vi "stopReading.vi"(8 "error in (no error)":errorcluster, 10 "Electrometer in":refnum<class "Electrometer.lvclass">, 11 "State in":refnum<class "State.lvclass">) -> (0 "error out":errorcluster, 2 "Electrometer out":refnum<class "Electrometer.lvclass">, 3 "State out":refnum<class "State.lvclass">)   [LabVIEW 2016, in "State.lvclass"]
uses:
  State.lvclass
  Electrometer.lvclass
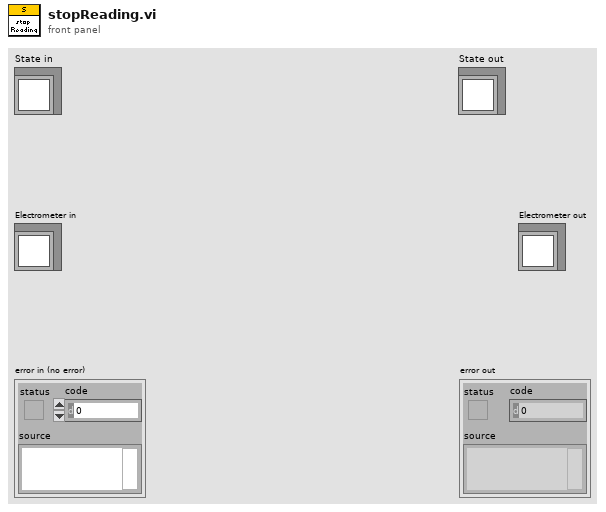
[diagram p1: front panel]
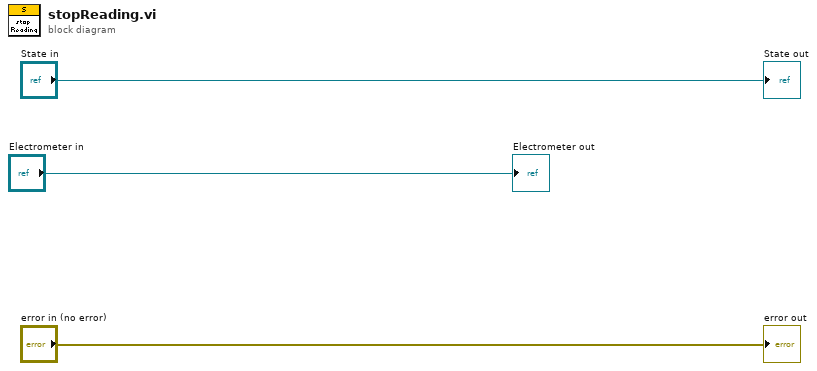
[diagram p0: block diagram]
diagram:
  "error out" <- "error in (no error)"
  "State out" <- "State in"
  "Electrometer out" <- "Electrometer in"
